vi "Log File Information.vi"(8 "error in (no error)":errorcluster, 9 "Log File Path":path, 10 "2nd Most Recent File Path":path, 11 "Most Recent File Path":path) -> (0 "error out":errorcluster)   [LabVIEW 2013]
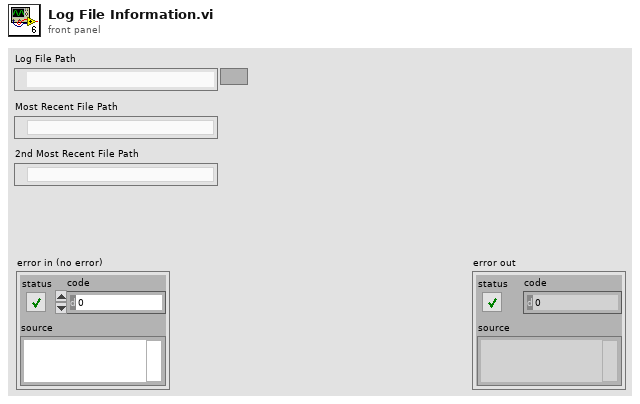
[diagram p1: front panel]
types:
  T1 = enum16{"open", "replace", "create", "open or create", "replace or create", "replace or create with confirmation"}
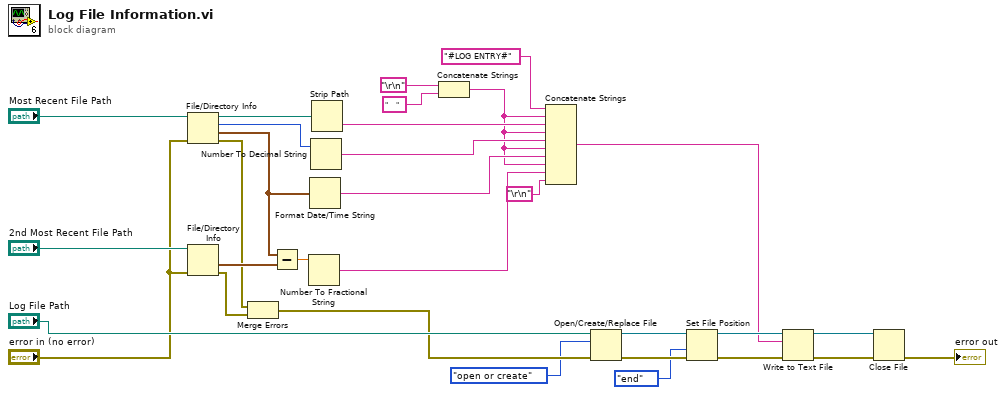
[diagram p0: block diagram]
diagram:
  n1 = File/Directory Info(path="Most Recent File Path", error in="error in (no error)") -> (path out=w21:path, size=w19:i64, last mod=w15:timestamp, error out=w11:errorcluster)  [unwired: 3 out]
  n2 = File/Directory Info(path="2nd Most Recent File Path", error in="error in (no error)") -> (last mod=w16:timestamp, error out=w13:errorcluster)  [unwired: 5 out]
  n3 = Merge Errors(w11, w13) -> (w12:errorcluster)
  n4 = Subtract(x=w15, y=w16) -> (x-y=w14:dbl)
  n5 = Number To Fractional String(number=w14) -> (F-format string=w7:string)  [unwired: 3 in]
  n6 = Format Date/Time String(seconds (now)=w15) -> (date/time string=w8:string)  [unwired: 2 in]
  n7 = Number To Decimal String(number=w19) -> (decimal integer string=w9:string)  [unwired: 1 in]
  n8 = Strip Path(path=w21) -> (name=w10:string)  [unwired: 1 out]
  n9 = Concatenate Strings("\r\n", "    " ("string")) -> (w2:string)
  n10 = Concatenate Strings("#LOG ENTRY#" ("string"), w2, w10, w2, w9, w2, w8, w2, w7, "\r\n") -> (w6:string)
  n11 = Open/Create/Replace File(file path (use dialog)="Log File Path", error in=w12, operation (0:open)=T1."open or create") -> (refnum out=w27:refnum<file>, error out=w28:errorcluster)  [unwired: 3 in, 1 out]
  n12 = Set File Position(refnum=w27, from (0:start)=enum16{"start", "end", "current"}."end", error in=w28) -> (refnum out=w24:refnum<file>, error out=w25:errorcluster)  [unwired: 1 in]
  n13 = Write to Text File(file (use dialog)=w24, text=w6, error in=w25) -> (refnum out=w22:refnum<file>, error out=w23:errorcluster)  [unwired: 1 in, 1 out]
  n14 = Close File(refnum=w22, error in=w23) -> (error out=→"error out":errorcluster)  [unwired: 1 out]
